vi "Handle Specific Message.vi"(11 "Handler in":refnum<class "Handler.lvclass">) -> ()   [LabVIEW 2024, in "Ramses Framework.lvlib" / "Handler.lvclass"]
uses:
  Handler.lvclass
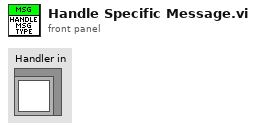
[diagram p1: front panel]
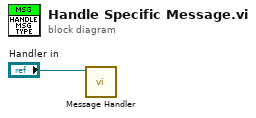
[diagram p0: block diagram]
diagram:
  n1 = call-dynamic "Message Handler.vi"("Message Handler in"="Handler in") -> ()  [unwired: 11 in]
